vi "GetExitEvent.vi"(8 "error in (no error)":errorcluster, 11 "ClassByRef in":refnum<class "ClassByRef.lvclass">) -> (0 "error out":errorcluster, 2 "ExitEvent":refnum<user-event>, 3 "ClassByRef out":refnum<class "ClassByRef.lvclass">)   [LabVIEW 2021, in "ClassUtilities.lvlib" / "ClassByRef.lvclass"]
uses:
  ClassByRef.lvclass
  ClassByRef.lvclass/ClassByRef.ctl
  d78f5ac1-b881-48f7-a86d-8a9fda2b8e49.vi
  GetRef.vi
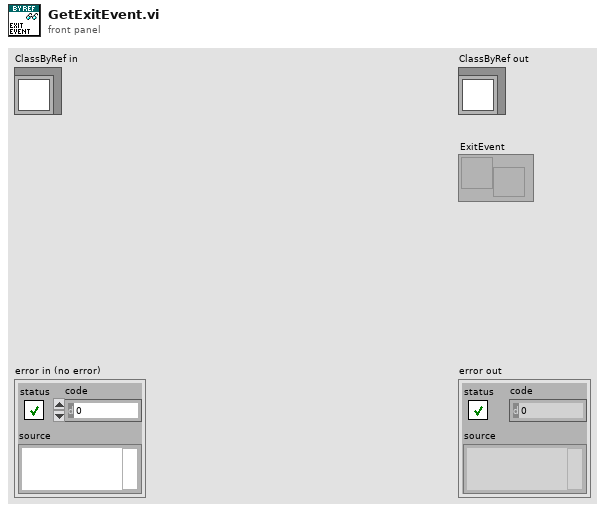
[diagram p1: front panel]
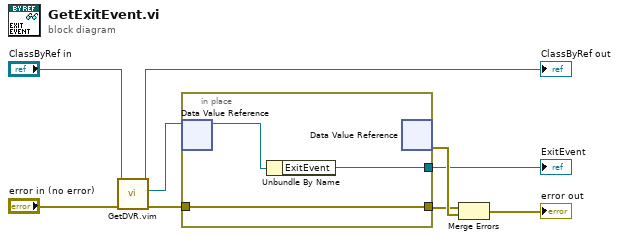
[diagram p0: block diagram]
diagram:
  n1 = call "GetDVR.vim"("error in (no error)"="error in (no error)", "ByRefClass in"="ClassByRef in") -> ("error out"=w3:errorcluster, "DVR"=w4:refnum<data-value>, "ByRefClass out"=→"ClassByRef out":refnum<class "ClassByRef.lvclass">)  [unwired: 7 in]
  n2 = in-place {
    in-place-border: w3 -> [w12]
    in-place-border: [w12] -> w7
    in-place-border: [w10] -> w1
    n3 = in-place-dvr #1(w4) -> (w11:refnum<class "ClassByRef.lvclass">)  [unwired: 1 out]
    n4 = Unbundle By Name(w11) -> ("ExitEvent"=w10:refnum<user-event>)
    n5 = in-place-dvr #1() -> (w8:errorcluster)  [unwired: 1 in, 1 out]
  }
  "ExitEvent" <- w1
  n6 = Merge Errors(w7, w8) -> (→"error out":errorcluster)
